vi "getLocalTravelAbove.vi"(7 "Exclude Array":T1[](array[typedef]) {"Sizes"."Min" format="%#.1f"; "Sizes"."Max" format="%#.1f"}, 10 "pointA":sgl[](array[numeric])) -> (2 "travelAboveHeight":sgl)   [LabVIEW 2021]
uses:
  Route mapping/Exclude_cluster.ctl
  Route mapping/Box_size.ctl
  Route mapping/Exclusion_type.ctl
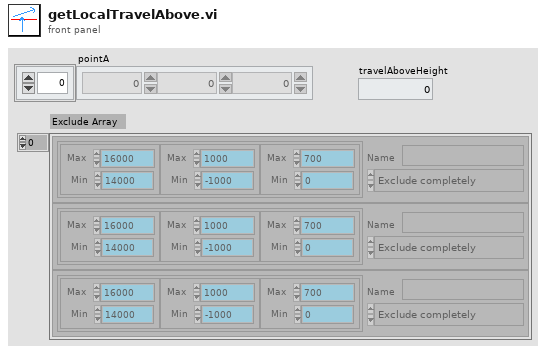
[diagram p1: front panel]
types:
  T1 = typedef "Exclude_cluster.ctl" = cluster{"Sizes":T2, "Name":string, "Exclude Type":T3}
  T2 = typedef "Box_size.ctl" = cluster{"Max":sgl, "Min":sgl}[]
  T3 = typedef "Exclusion_type.ctl" = enum16{"Exclude completely", "Allow only vertical moves"}
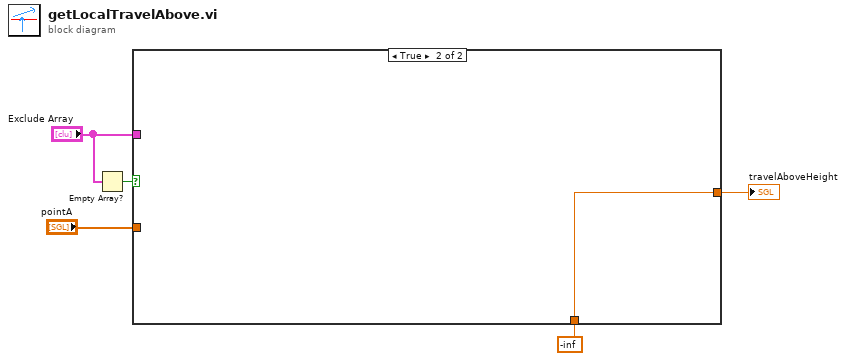
[diagram p0: block diagram]
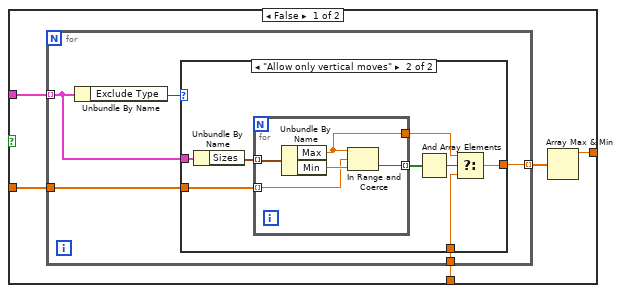
[diagram p2: hidden frame]
diagram:
  n1 = Empty Array?(array="Exclude Array") -> (empty?=w2:bool)
  n2 = case shown="True" w2 {
    tunnel: "pointA" -> [w10 _]
    tunnel: sgl -inf ("f") -> [w9 w30]
    tunnel: [w7 w30] -> w3
    tunnel: "Exclude Array" -> [w6 _]
    frame False {
      n3 = for {
        tunnel: w6 -> [w14] mode=indexing
        tunnel: w10 -> [w15]
        tunnel: w9 -> [w12]
        tunnel: [w11] -> w8 mode=indexing
        n4 = Unbundle By Name(w14) -> ("Exclude Type"=w13:T3)
        n5 = case shown="\"Allow only vertical moves\"" w13 {
          tunnel: w15 -> [_ w23]
          tunnel: w14 -> [_ w21]
          tunnel: w12 -> [w16 w18]
          tunnel: [w16 w17] -> w11
          frame "Exclude completely", Default {
          }
          frame "Allow only vertical moves" {
            n6 = Unbundle By Name(w21) -> ("Sizes"=w24:T2)
            n7 = for {
              tunnel: w24 -> [w29] mode=indexing
              tunnel: w23 -> [w27] mode=indexing
              tunnel: [w26] -> w22 mode=indexing
              tunnel: [w25] -> w19
              n8 = Unbundle By Name(w29) -> ("Max"=w25:sgl, "Min"=w28:sgl)
              n9 = In Range and Coerce(upper limit=w25, x=w27, lower limit=w28) -> (In Range?=w26:bool)  [unwired: 1 out]
            }
            n10 = And Array Elements(Boolean array=w22) -> (logical AND=w20:bool)
            n11 = Select(t=w19, s=w20, f=w18) -> (s? t:f=w17:sgl)
          }
        }
      }
      n12 = Array Max & Min(array=w8) -> (max value=w7:sgl)  [unwired: 3 out]
    }
    frame True {
    }
  }
  "travelAboveHeight" <- w3
